vi "启动-报警记录预览窗口.vi"(8 "错误输入（无错误）":errorcluster, 11 "报警数据缓存文件":path) -> (0 "error out":errorcluster caption="错误输出")   [LabVIEW 2017]
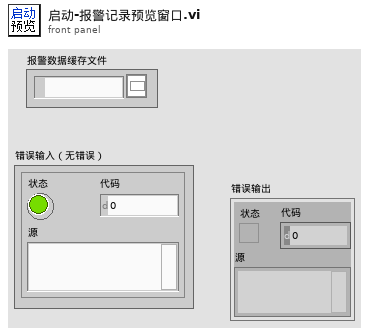
[diagram p1: front panel]
types:
  T1 = enum32{"Invalid", "Standard", "Closed", "Hidden", "Minimized", "Maximized"}
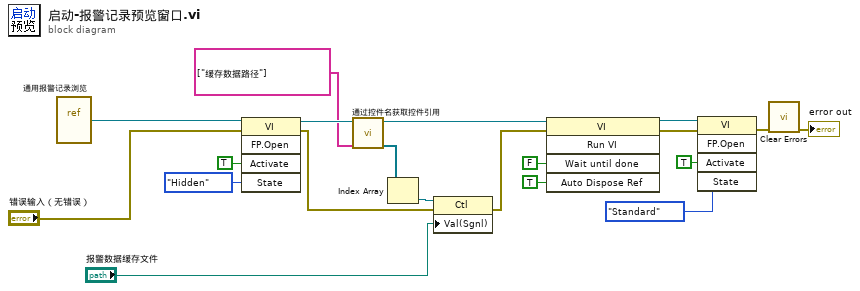
[diagram p0: block diagram]
diagram:
  n1 = vi-ref "通用报警记录浏览.vi"() -> (w20:refnum<vi>)
  n2 = invoke class="VI" method="FP.Open"(reference=w20, error in="错误输入（无错误）", "Activate"=TRUE ("激活？"), "State"=T1."Hidden" ("状态")) -> (reference out=w16:refnum<vi>, error out=w4:errorcluster)  [unwired: 1 in, 3 out]
  n3 = call "通过控件名获取控件引用.vi"("控件名数组"=string[] ["缓存数据路径"], "VI引用"=w16) -> ("控件引用输出"=w14:refnum<vi>[], "VI引用o"=w12:refnum<vi>)  [unwired: 7 in, 1 out]
  n4 = Index Array(array=w14) -> (element=w13:refnum<vi>)  [unwired: 1 in]
  n5 = property class="Ctl"(reference=w13, error in=w4, "Val(Sgnl)"="报警数据缓存文件") -> (error out=w3:errorcluster)  [unwired: 1 out]
  n6 = invoke class="VI" method="Run VI"(reference=w12, error in=w3, "Wait until done"=FALSE ("结束前等待"), "Auto Dispose Ref"=TRUE ("自动销毁引用")) -> (reference out=w9:refnum<vi>, error out=w8:errorcluster)  [unwired: 1 in, 3 out]
  n7 = invoke class="VI" method="FP.Open"(reference=w9, error in=w8, "Activate"=TRUE ("激活？"), "State"=T1."Standard" ("状态")) -> (error out=w5:errorcluster)  [unwired: 1 in, 4 out]
  n8 = call <vilib>:"Clear Errors.vi"("error in (no error)"=w5) -> ("error out"=→"error out":errorcluster)  [unwired: 5 in, 1 out]
